vi "Create Device.vi"(8 "Error In":errorcluster, 10 "Devices":i32, 11 "Platform Names":i32) -> (0 "error out":errorcluster, 3 "Device Reference":T1)   [LabVIEW 2012, in "OpenCLV x64.lvlib"]
doc: "Creates a new OpenCLV device that that is required before using any other OpenCLV commands."
uses:
  OpenCLV x64.lvlib
  Controls/Device ID.ctl
  Error Checking/Add Error Functional Global.vi
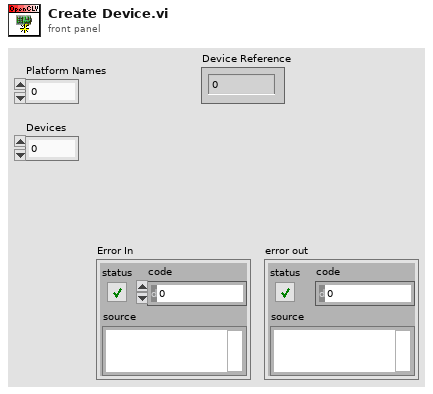
[diagram p1: front panel]
types:
  T1 = typedef "OpenCLV x64.lvlib/Device ID.ctl" = u64
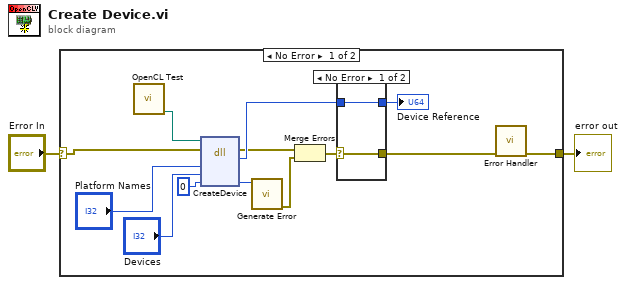
[diagram p0: block diagram]
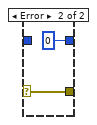
[diagram p2: hidden frame]
diagram:
  n1 = case shown="No Error" "Error In" {
    selector: "Error In" -> [w3 w20]
    tunnel: [w7 w20] -> w2
    frame No Error {
      n2 = call "OpenCL Test.vi"() -> ("DLL To Use"=w10:path)  [unwired: 11 in]
      n3 = dll-call lib="C:/Users/bme-amcelroy-la/Desktop/OpenCLV/trunk/OpenCLV_x64_1.0/OpenCLV_x64.dll" fn="CreateDevice"(path in=w10, error in=w3, "Platform ID"="Platform Names", "Device ID"="Devices", "Error"=0) -> (error out=w5:errorcluster, "Device Reference"=w13:u64, "Error"=w12:i32)  [unwired: 3 in, 1 out]
      n4 = call "Generate Error.vi"("Error"=w12) -> ("error out"=w6:errorcluster)  [unwired: 10 in]
      n5 = Merge Errors(w5, w6) -> (w4:errorcluster)
      n6 = case shown="No Error" w4 {
        selector: w4 -> [w16 w19]
        tunnel: w13 -> [w17 _]
        tunnel: [w16 w19] -> w8
        tunnel: [w17 u64 0 ("Device Reference")] -> w9
        frame No Error {
        }
        frame Error {
        }
      }
      "Device Reference" <- w9
      n7 = call-poly "Error Handler.vi"("Error In"=w8) -> ("Error Out"=w7:errorcluster)  [unwired: 10 in]
    }
    frame Error {
    }
  }
  "error out" <- w2
